vi "HIOKI PW3390 Conf Measure Item sub3.vi"(1 "Integrate":T1) -> (0 "Integrate out":bool[][](array[boolean]))   [LabVIEW 2009]
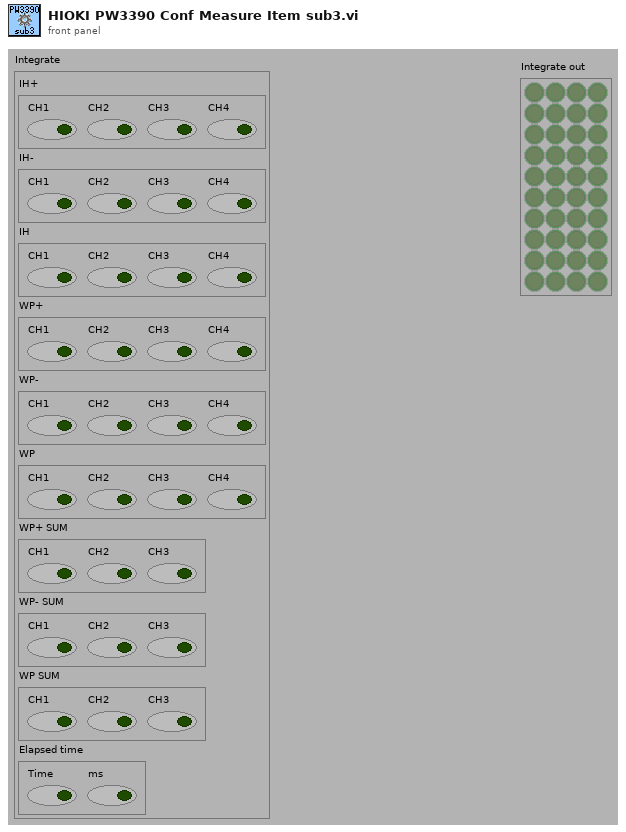
[diagram p1: front panel]
types:
  T1 = cluster{"IH+":cluster{"CH1":bool, "CH2":bool, "CH3":bool, "CH4":bool}, "IH-":cluster{"CH1":bool, "CH2":bool, "CH3":bool, "CH4":bool}, "IH":cluster{"CH1":bool, "CH2":bool, "CH3":bool, "CH4":bool}, "WP+":cluster{"CH1":bool, "CH2":bool, "CH3":bool, "CH4":bool}, "WP-":cluster{"CH1":bool, "CH2":bool, "CH3":bool, "CH4":bool}, "WP":cluster{"CH1":bool, "CH2":bool, "CH3":bool, "CH4":bool}, "WP+ SUM":cluster{"CH1":bool, "CH2":bool, "CH3":bool}, "WP- SUM":cluster{"CH1":bool, "CH2":bool, "CH3":bool}, "WP SUM":cluster{"CH1":bool, "CH2":bool, "CH3":bool}, "Elapsed time":cluster{"Time":bool, "ms":bool}}
  T2 = cluster{"CH1":bool, "CH2":bool, "CH3":bool, "CH4":bool}
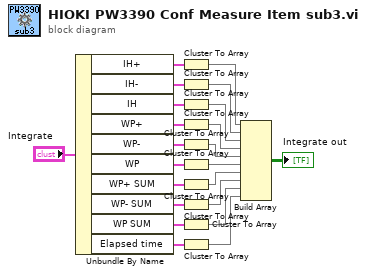
[diagram p0: block diagram]
diagram:
  n1 = Unbundle By Name("Integrate") -> ("IH+"=w17:T2, "IH-"=w16:T2, "IH"=w15:T2, "WP+"=w14:T2, "WP-"=w13:T2, "WP"=w12:T2, "WP+ SUM"=w11:cluster{"CH1":bool, "CH2":bool, "CH3":bool}, "WP- SUM"=w10:cluster{"CH1":bool, "CH2":bool, "CH3":bool}, "WP SUM"=w9:cluster{"CH1":bool, "CH2":bool, "CH3":bool}, "Elapsed time"=w8:cluster{"Time":bool, "ms":bool})
  n2 = Cluster To Array(cluster=w17) -> (array=w19:bool[])
  n3 = Cluster To Array(cluster=w16) -> (array=w20:bool[])
  n4 = Cluster To Array(cluster=w15) -> (array=w21:bool[])
  n5 = Cluster To Array(cluster=w14) -> (array=w7:bool[])
  n6 = Cluster To Array(cluster=w13) -> (array=w6:bool[])
  n7 = Cluster To Array(cluster=w12) -> (array=w5:bool[])
  n8 = Cluster To Array(cluster=w11) -> (array=w4:bool[])
  n9 = Cluster To Array(cluster=w10) -> (array=w3:bool[])
  n10 = Cluster To Array(cluster=w9) -> (array=w2:bool[])
  n11 = Cluster To Array(cluster=w8) -> (array=w1:bool[])
  n12 = Build Array(w19, w20, w21, w7, w6, w5, w4, w3, w2, w1) -> (→"Integrate out":bool[][])
